vi "Create Master Station.vi"(5 "error in":errorcluster, 7 "Session Cluster":T1={"Source"=3, "Destination"=4}, 8 "Channel Cluster":T2) -> (0 "error out":errorcluster, 1 "DNP3 master":refnum<k21>, 2 "DNP3 channel":refnum<k21>, 3 "DNP3 master session":refnum<k21>)   [LabVIEW 2016]
doc: "Creates a master station and configures the channel and session settings."
uses:
  channnel_setting_Master.ctl
  session_setting_Master.ctl
  <vilib>/DNP3/DNP3_Master/Create Master Serial Channel.vi
  <vilib>/DNP3/DNP3_Master/Create Master IP Channel.vi
  <vilib>/DNP3/DNP3_Master.lvlib
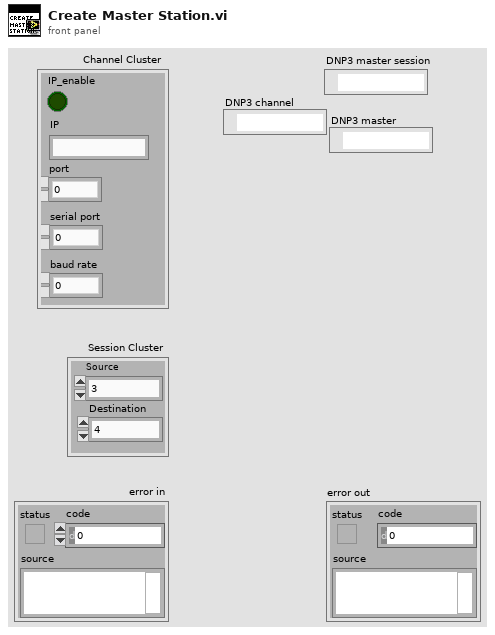
[diagram p1: front panel]
types:
  T1 = typedef "session_setting_Master.ctl" = cluster{"Source":u16, "Destination":u16}
  T2 = typedef "channnel_setting_Master.ctl" = cluster{"IP_enable":bool, "IP":string, "port":u16, "serial port":u16, "baud rate":u32}
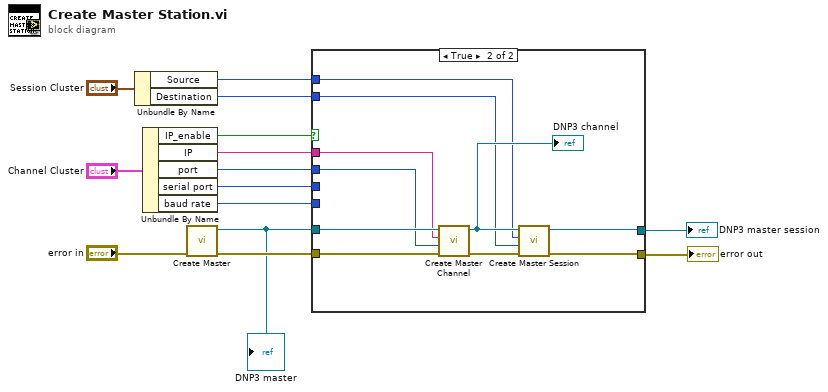
[diagram p0: block diagram]
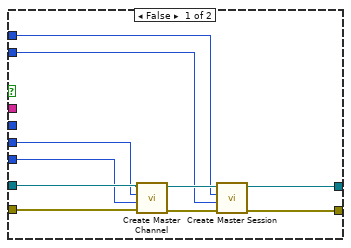
[diagram p2: hidden frame]
diagram:
  n1 = Unbundle By Name("Session Cluster") -> ("Source"=w6:u16, "Destination"=w5:u16)
  n2 = Unbundle By Name("Channel Cluster") -> ("IP_enable"=w13:bool, "IP"=w8:string, "port"=w7:u16, "serial port"=w2:u16, "baud rate"=w1:u32)
  n3 = call <vilib>:"Create Master.vi"("error in (no error)"="error in") -> ("error out"=w10:errorcluster, "DNP3 master"=w9:refnum<k21>)  [unwired: 9 in]
  "DNP3 master" <- w9
  n4 = case shown="True" w13 {
    tunnel: w10 -> [w23 w34]
    tunnel: w9 -> [w22 w32]
    tunnel: w8 -> [_ w28]
    tunnel: w7 -> [_ w27]
    tunnel: w6 -> [w20 w26]
    tunnel: w5 -> [w19 w25]
    tunnel: [w18 w30] -> w4
    tunnel: [w17 w29] -> w3
    tunnel: w2 -> [w16 _]
    tunnel: w1 -> [w15 _]
    frame False {
      n5 = call-poly <vilib>:"Create Master Channel.vi"("error in (no error)"=w23, "baud rate (9600)"=w15, "serial port"=w16, "DNP3 master"=w22) -> ("error out"=w24:errorcluster, "DNP3 channel"=w21:refnum<k21>)  [unwired: 6 in]
      n6 = call <vilib>:"Create Master Session.vi"("error in (no error)"=w24, "destination"=w19, "source"=w20, "DNP3 channel"=w21) -> ("error out"=w17:errorcluster, "DNP3 master session"=w18:refnum<k21>)  [unwired: 6 in]
    }
    frame True {
      n7 = call-poly <vilib>:"Create Master Channel.vi"("error in (no error)"=w34, "port (20000)"=w27, "IP"=w28, "DNP3 master"=w32) -> ("error out"=w33:errorcluster, "DNP3 channel"=w31:refnum<k21>)  [unwired: 6 in]
      "DNP3 channel" <- w31
      n8 = call <vilib>:"Create Master Session.vi"("error in (no error)"=w33, "destination"=w25, "source"=w26, "DNP3 channel"=w31) -> ("error out"=w29:errorcluster, "DNP3 master session"=w30:refnum<k21>)  [unwired: 6 in]
    }
  }
  "error out" <- w3
  "DNP3 master session" <- w4
